vi "VerifyArguments.vi"(8 "error in (no error)":errorcluster, 11 "MassCompile in":refnum<class "MassCompile.lvclass">) -> (0 "error out":errorcluster, 3 "MassCompile out":refnum<class "MassCompile.lvclass">)   [LabVIEW 2014, in "MassCompile.lvclass"]
uses:
  MassCompile.lvclass
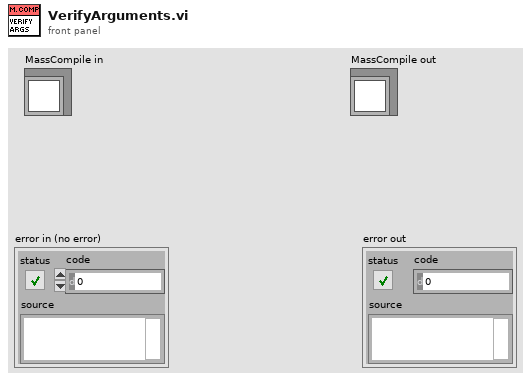
[diagram p1: front panel]
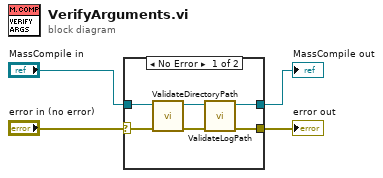
[diagram p0: block diagram]
diagram:
  n1 = case shown="No Error" "error in (no error)" {
    selector: "error in (no error)" -> [w10 w12]
    tunnel: [w7 w12] -> w2
    tunnel: [w9 w11] -> w1
    tunnel: "MassCompile in" -> [w6 w11]
    frame No Error {
      n2 = call "ValidateDirectoryPath.vi"("error in (no error)"=w10, "MassCompile in"=w6) -> ("error out"=w8:errorcluster, "MassCompile out"=w5:refnum<class "MassCompile.lvclass">)  [unwired: 8 in]
      n3 = call "ValidateLogPath.vi"("error in (no error)"=w8, "MassCompile in"=w5) -> ("error out"=w7:errorcluster, "MassCompile out"=w9:refnum<class "MassCompile.lvclass">)  [unwired: 8 in]
    }
    frame Error {
    }
  }
  "error out" <- w2
  "MassCompile out" <- w1
